vi "Out_S5F4.vi"(8 "error in (no error)":errorcluster, 11 "S5 Message Class in":refnum<class "S5 Message Class.lvclass">) -> (0 "error out":errorcluster, 3 "S5 Message Class out":refnum<class "S5 Message Class.lvclass">)   [LabVIEW 2020, in "SECS Communication.lvlib" / "S5 Message Class.lvclass"]
uses:
  S5 Message Class.lvclass
  D:/Dropbox/SECS/SECS_GEM v1.0.6/Com/SECS Communication/SECS-II Class/SECS-II Class.lvclass
  SECS-II Class/Data Message_Binary.vi
  SECS-II Class/SECS-II Class.lvclass
  D:/Dropbox/SECS/SECS_GEM v1.0.6/Com/SECS Communication/S5 Message Class/S5 Message Class.lvclass
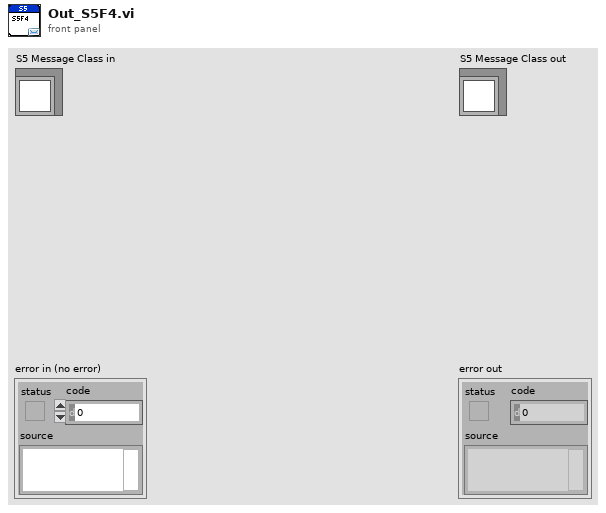
[diagram p1: front panel]
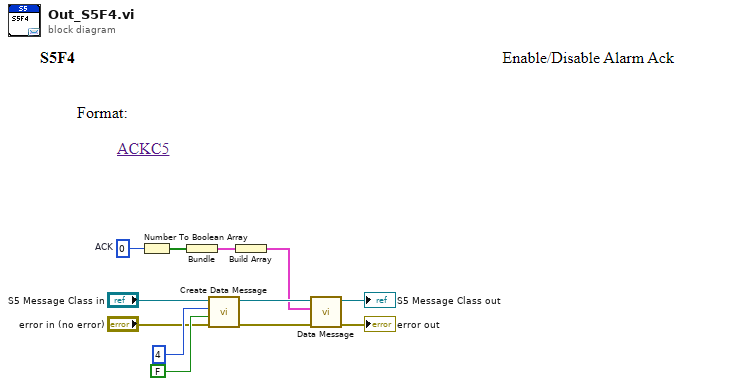
[diagram p0: block diagram]
diagram:
  w4 = u8 0  # ACK
  n1 = Number To Boolean Array(number=w4) -> (Boolean array=w3:bool[])
  n2 = Bundle("Boolean array"=w3) -> (w2:cluster{"Boolean array":bool[]})  [unwired: 1 in]
  n3 = call "Create Data Message.vi"("error in (no error)"="error in (no error)", "W-Bit"=FALSE, "Function"=u8 4, "SECS-II Class in"="S5 Message Class in") -> ("error out"=w10:errorcluster, "SECS-II Class out"=w9:refnum<class "S5 Message Class.lvclass">)  [unwired: 6 in]
  n4 = Build Array(w2) -> (w1:cluster{"Boolean array":bool[]}[])
  n5 = call-poly "Data Message.vi"("error in"=w10, "Data Cluster"=w1, "SECS-II Class in"=w9) -> ("error out"=→"error out":errorcluster, "SECS-II Class out"=→"S5 Message Class out":refnum<class "S5 Message Class.lvclass">)  [unwired: 7 in]
